vi "DMM Measure Voltage.vi"(6 "Timeout (5000 milliseconds)":u32=1000, 8 "error in (no error)":errorcluster, 9 "Sample Count (1)":i32=1, 10 "Channel List (101:110)":string="107", 11 "DMM":refnum<visa-resource-name>="COM1") -> (0 "error out":errorcluster, 1 "Voltage":dbl format="%0.8f", 2 "Voltage Data":dbl[](array[numeric]))   [LabVIEW 2015]
uses:
  <instrlib>/Keithley 27XX/Public/Data/Read Multiple Direct.vi
  <instrlib>/Keithley 27XX/Keithley 27XX.lvlib
panel:
  in  "Enable Auto Range (True)":bool=TRUE
  in  "Serial Configuration":T1={"Baud Rate (19200)"=19200, "Flow Control (1: XON/XOFF)"=1, "Termination Char (0:CR)"=0} {"Termination Char (0:CR)" items=["CR", "LF"]; "Flow Control (1: XON/XOFF)" items=["None", "XON/XOFF", "RTS/CTS (2701 Only)", "XON/XOFF & RTS/CTS (2701 Only)"]; "Baud Rate (19200)" items=["300"=300, "600"=600, "1200"=1200, "2400"=2400, "4800"=4800, "9600"=9600, "19.2k"=19200, "38.4k (2701 Only)"=38400, "57.6k (2701 Only)"=57600, "115.2k (2701 Only)"=115200]}
  in  "Function (0: DC Voltage)":u16(ring) items=["DC Voltage", "AC Voltage", "DC Current", "AC Current", "Resistance", "Four-Wire Resistance", "Temperature (C)", "Frequency", "Period", "Continuity"]
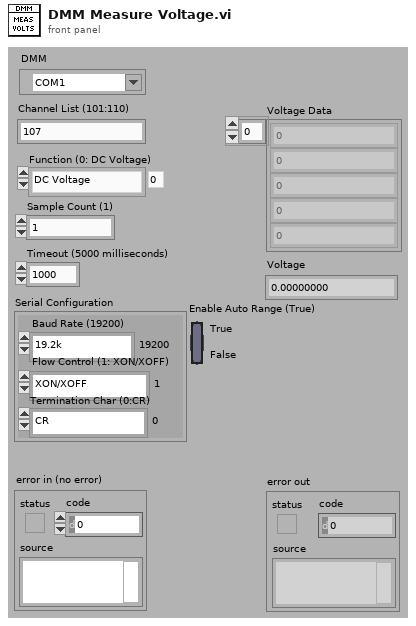
[diagram p1: front panel]
types:
  T1 = cluster{"Baud Rate (19200)":u32, "Flow Control (1: XON/XOFF)":u16, "Termination Char (0:CR)":u16}
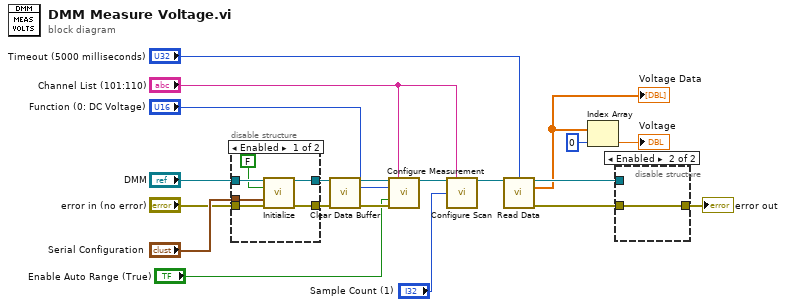
[diagram p0: block diagram]
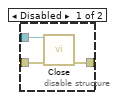
[diagram p3: hidden frame]
diagram:
  n1 = disable-structure shown="Enabled" {
    disable-tunnel: [w26 _] -> w15
    disable-tunnel: [w25 w27] -> w14
    disable-tunnel: "Serial Configuration" -> [w24 _]
    disable-tunnel: "error in (no error)" -> [w23 _]
    disable-tunnel: "DMM" -> [w22 w27]
    frame Enabled {
      n2 = call <instrlib>:"Initialize.vi"("VISA resource name"=w22, "ID Query? (T: Yes)"=FALSE, "Serial Configuration"=w24, "error in (no error)"=w23) -> ("VISA resource name out"=w25:refnum<visa-resource-name>, "error out"=w26:errorcluster)  [unwired: 10 in]
    }
    frame Disabled {
    }
  }
  n3 = call <instrlib>:"Clear Data Buffer.vi"("VISA resource name"=w14, "error in (no error)"=w15) -> ("VISA resource name out"=w17:refnum<visa-resource-name>, "error out"=w16:errorcluster)  [unwired: 12 in]
  n4 = call <instrlib>:"Configure Measurement.vi"("VISA resource name"=w17, "Scan List (Empty)"="Channel List (101:110)", "Function (0: DC Voltage)"="Function (0: DC Voltage)", "Enable Auto Range (True)"="Enable Auto Range (True)", "error in (no error)"=w16) -> ("VISA resource name out"=w20:refnum<visa-resource-name>)  [unwired: 9 in, 1 out]
  n5 = call <instrlib>:"Configure Scan.vi"("VISA resource name"=w20, "Channel List (101:110)"="Channel List (101:110)", "Sample Count (100)"="Sample Count (1)") -> ("VISA resource name out"=w12:refnum<visa-resource-name>)  [unwired: 11 in, 1 out]
  n6 = call-poly <instrlib>:"Read Data.vi"("VISA resource name"=w12, "Timeout (30000 milliseconds)"="Timeout (5000 milliseconds)") -> ("VISA resource name out"=w19:refnum<visa-resource-name>, "Measurement Data"=w7:dbl[], "error out"=w18:errorcluster)  [unwired: 8 in, 3 out]
  "Voltage Data" <- w7
  n7 = Index Array(array=w7, index=0) -> (element=→"Voltage":dbl)
  n8 = disable-structure shown="Enabled" {
    disable-tunnel: w19 -> [w30 _]
    disable-tunnel: w18 -> [w29 w31]
    disable-tunnel: [w28 w31] -> w5
    frame Disabled {
      n9 = call <instrlib>:"Close.vi"("VISA resource name"=w30, "error in (no error)"=w29) -> ("error out"=w28:errorcluster)  [unwired: 13 in]
    }
    frame Enabled {
    }
  }
  "error out" <- w5
